vi "PSK.vi"() -> ()   [LabVIEW 2013]
panel:
  out "Waveform Graph":dynamicdata(graph)
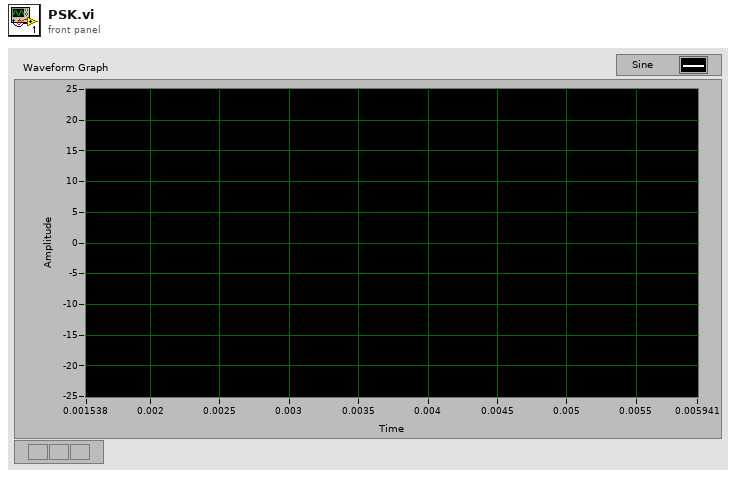
[diagram p1: front panel]
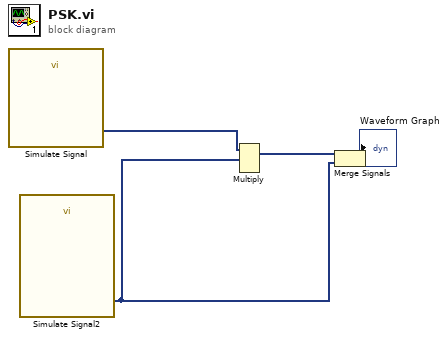
[diagram p0: block diagram]
diagram:
  n1 = call "Simulate Signal"() -> ("Sine"=w4:dynamicdata)  [unwired: 14 in, 1 out]
  n2 = call "Simulate Signal2"() -> ("Square"=w1:dynamicdata)  [unwired: 14 in, 1 out]
  n3 = Multiply(1:w1, 2:w4) -> (0:w3:dynamicdata)  [unwired: 1 in, 1 out]
  n4 = Merge Signals(w3, w1) -> (→"Waveform Graph":dynamicdata)
